vi "Write Command Name.vi"(8 "error in (no error)":errorcluster, 10 "Name":string, 11 "Command in":refnum<class "Command State Actor.lvclass">) -> (0 "error out":errorcluster, 3 "Command out":refnum<class "Command State Actor.lvclass">)   [LabVIEW 2013, in "Command State Actor.lvlib" / "Command State Actor.lvclass"]
uses:
  Command State Actor.lvclass
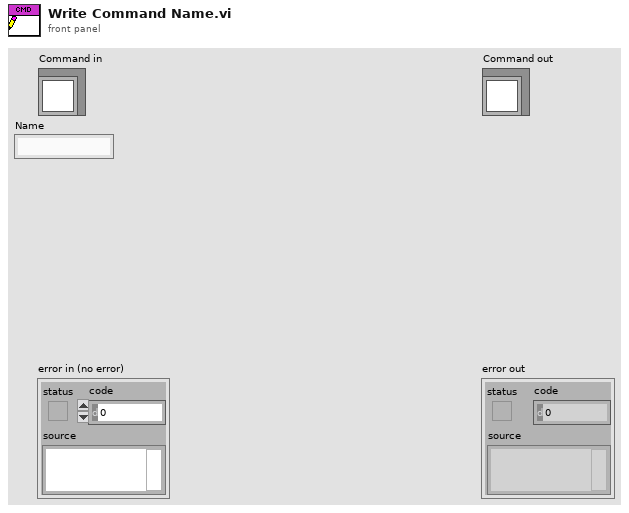
[diagram p1: front panel]
types:
  T1 = typedef "Command State Actor.lvlib/Command State Actor.lvclass/Command Status.ctl" = cluster{"CurrentCommandState":T2, "Command Name":string, "Current State Status":T3, "Command Start Time":timestamp, "Command End Time":timestamp, "Previous State Status":T3}
  T2 = typedef "Command State Actor.lvlib/Command State Actor.lvclass/Command States.ctl" = enum16{"NotStarted", "Starting", "Started", "Executing", "Completing", "Completed", "Stopping", "Stopped"}
  T3 = typedef "Command Actor.lvlib/Command States.lvclass/State Status.ctl" = cluster{"State Name":string, "State Entry Time":timestamp, "State Exit Time":timestamp}
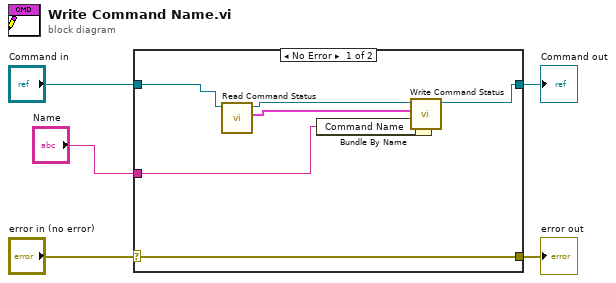
[diagram p0: block diagram]
diagram:
  n1 = case shown="No Error" "error in (no error)" {
    selector: "error in (no error)" -> [w12 w13]
    tunnel: [w12 w13] -> w4
    tunnel: [w9 w14] -> w2
    tunnel: "Command in" -> [w11 w14]
    tunnel: "Name" -> [w6 _]
    frame No Error {
      n2 = call-dynamic "Read Command Status.vi"("Command in"=w11) -> ("Command Status"=w8:T1, "Command out"=w10:refnum<class "Command State Actor.lvclass">)  [unwired: 8 in, 1 out]
      n3 = Bundle By Name(cluster=w8, "Command Name"=w6) -> (w7:T1)
      n4 = call-dynamic "Write Command Status.vi"("Command Status"=w7, "Command in"=w10) -> ("Command out"=w9:refnum<class "Command State Actor.lvclass">)  [unwired: 8 in, 1 out]
    }
    frame Error {
    }
  }
  "error out" <- w4
  "Command out" <- w2
